vi "Initialise the Error log.vi"(8 "error in (no error)":errorcluster, 10 "Schema":string, 11 "Error Log in":refnum<class "Error Log.lvclass">) -> (0 "error out":errorcluster, 3 "Error Log out":refnum<class "Error Log.lvclass">)   [LabVIEW 2023, in "Data Analysis.lvlib" / "Error Log.lvlib" / "Error Log.lvclass"]
uses:
  Error Log.lvclass
  Error Log.lvclass/Error Log.ctl
  HardwareAbstractionLayer_LVOOP/Database/Database.lvclass
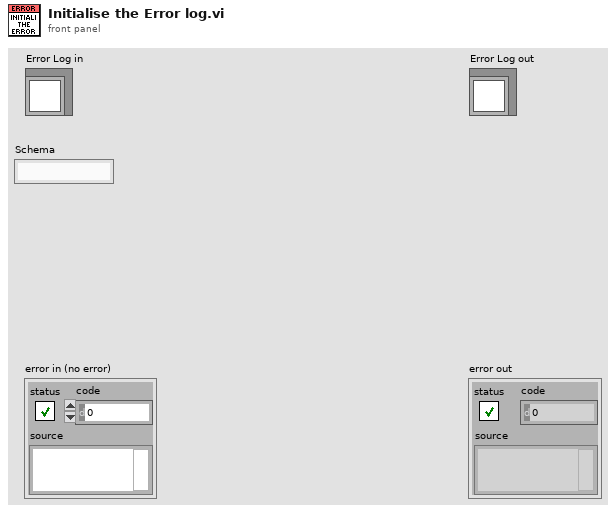
[diagram p1: front panel]
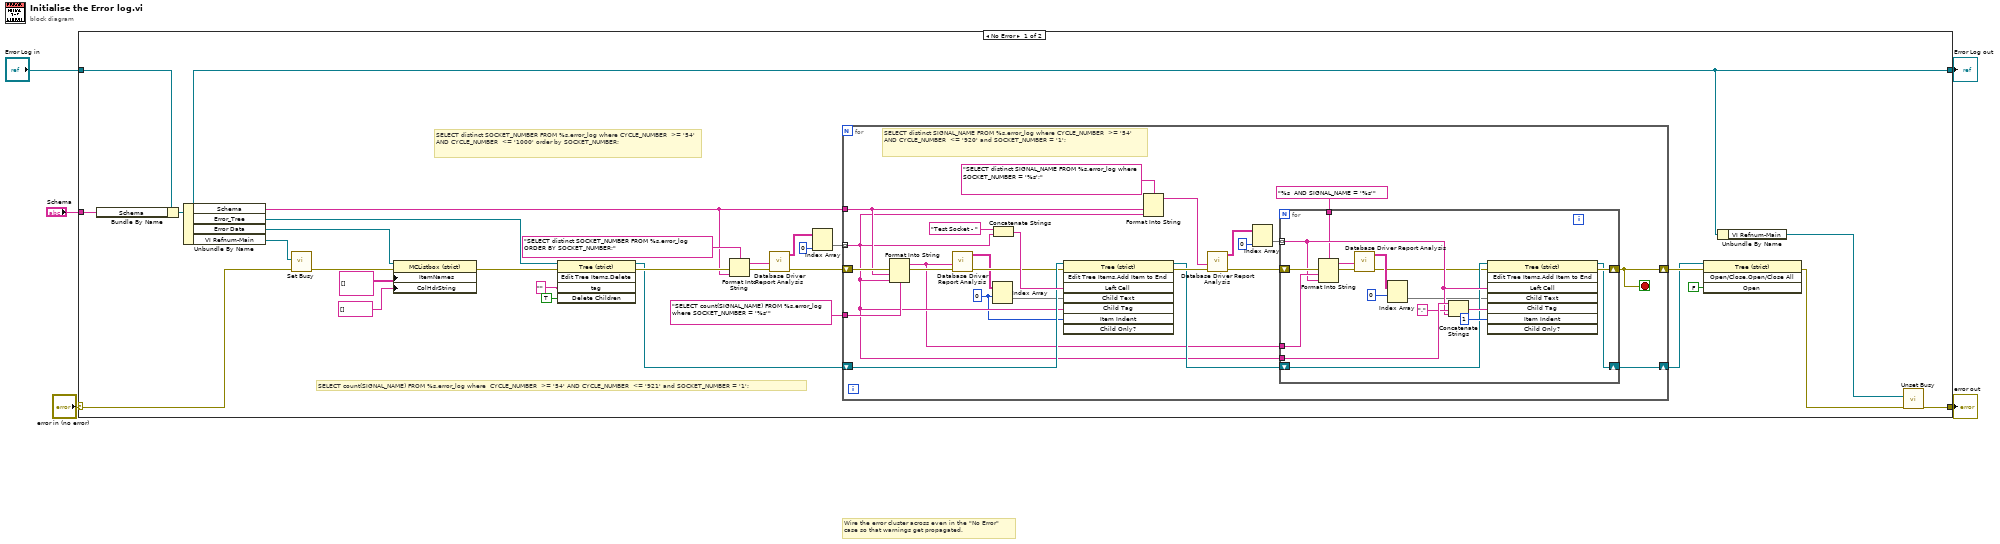
[diagram p0: block diagram]
diagram:
  # "Wire the error cluster across even in the \"No Error\"\ncase so that warnings get propagated."
  n1 = case shown="No Error" "error in (no error)" {
    selector: "error in (no error)" -> [w11 w78]
    tunnel: [w9 w77] -> w3
    tunnel: "Error Log in" -> [w19 w77]
    tunnel: "Schema" -> [w18 _]
    tunnel: [w6 w78] -> w1
    frame No Error {
      # "SELECT count(SIGNAL_NAME) FROM %s.error_log where  CYCLE_NUMBER  >= '54' AND CYCLE_NUMBER  <= '921' and SOCKET_NUMBER = '1';"
      # "SELECT distinct SOCKET_NUMBER FROM %s.error_log where CYCLE_NUMBER  >= '54' AND CYCLE_NUMBER  <= '1000' order by SOCKET_NUMBER;"
      n2 = Bundle By Name(cluster=w19, "Schema"=w18) -> (w9:refnum<class "Error Log.lvclass">)
      n3 = Unbundle By Name(w9) -> ("Schema"=w17:string, "Error_Tree"=w20:refnum<vi>, "Error Data"=w16:refnum<vi>, "VI Refnum-Main"=w12:refnum<vi>)
      n4 = call <vilib>:"Set Busy.vi"("error in (no error)"=w11, "VI reference (current VI)"=w12) -> ("error out"=w10:errorcluster)  [unwired: 8 in, 1 out]
      n5 = property class="MCListbox (strict)"(reference=w16, error in=w10, "ItemNames"=string[][] [] ("Item Names"), "ColHdrString"=string[] [] ("Column Header Strings[]")) -> (error out=w13:errorcluster)  [unwired: 1 out]
      n6 = invoke on="Invoke Node" class="Tree (strict)" method="Edit Tree Items.Delete"(reference=w20, error in=w13, "tag"="" ("Tag"), "Delete Children"=TRUE ("Delete Children?")) -> (reference out=w21:refnum<vi>, error out=w33:errorcluster)  [unwired: 1 in, 3 out]
      n7 = Format Into String(format string="SELECT distinct SOCKET_NUMBER FROM %s.error_log ORDER BY SOCKET_NUMBER;" ("SQL query"), error in=w33, w17) -> (resulting string=w30:string, error out=w34:errorcluster)  [unwired: 1 in]
      n8 = call "Database Driver Report Analysis.vi"("error in"=w34, "SQL query"=w30) -> ("error out"=w26:errorcluster, "data"=w27:string[][])  [unwired: 6 in, 2 out]
      n9 = Index Array(array=w27, index (col)=0 ("disabled index (col)")) -> (element=w28:string[])  [unwired: 1 in]
      n10 = for {
        tunnel: w28 -> [w41] mode=indexing
        shift-right: [w57] -> w35
        shift-left: w26 -> [w45]
        tunnel: w17 -> [w42]
        shift-right: [w47] -> w23
        shift-left: w21 -> [w49]
        tunnel: "SELECT count(SIGNAL_NAME) FROM %s.error_log where SOCKET_NUMBER = '%s'" ("SQL query") -> [w43]
        stop <- w57 stop-if-true
        w38 = 0 ("index (row)")
        # "SELECT distinct SIGNAL_NAME FROM %s.error_log where CYCLE_NUMBER  >= '54' AND CYCLE_NUMBER  <= '920' and SOCKET_NUMBER = '1';"
        n11 = Format Into String(format string=w43, error in=w45, w42, w41) -> (resulting string=w37:string, error out=w44:errorcluster)  [unwired: 1 in]
        n12 = call "Database Driver Report Analysis.vi"("error in"=w44, "SQL query"=w37) -> ("error out"=w46:errorcluster, "data"=w40:string[][])  [unwired: 6 in, 2 out]
        n13 = Index Array(array=w40, index (row)=w38) -> (element=w39:string[])  [unwired: 1 in]
        n14 = Concatenate Strings("Test Socket - " ("element"), w41) -> (w58:string)
        n15 = invoke on="Invoke Node" class="Tree (strict)" method="Edit Tree Items.Add Item to End"(reference=w49, error in=w46, "Left Cell"=w58, "Child Text"=w39, "Child Tag"=w41, "Item Indent"=w38) -> (reference out=w48:refnum<vi>, error out=w56:errorcluster)  [unwired: 2 in, 6 out]
        n16 = Format Into String(format string="SELECT distinct SIGNAL_NAME FROM %s.error_log where SOCKET_NUMBER = '%s';" ("SQL query"), w42, w41) -> (resulting string=w53:string)  [unwired: 2 in, 1 out]
        n17 = call "Database Driver Report Analysis.vi"("error in"=w56, "SQL query"=w53) -> ("error out"=w55:errorcluster, "data"=w51:string[][])  [unwired: 6 in, 2 out]
        n18 = Index Array(array=w51, index (col)=0 ("disabled index (col)")) -> (element=w50:string[])  [unwired: 1 in]
        n19 = for {
          shift-right: [w76] -> w57
          shift-left: w55 -> [w70]
          tunnel: w50 -> [w68] mode=indexing
          tunnel: w41 -> [w74]
          shift-right: [w71] -> w47
          shift-left: w48 -> [w66]
          tunnel: w37 -> [w69]
          tunnel: "%s  AND SIGNAL_NAME = '%s'" ("format string") -> [w67]
          n20 = Format Into String(format string=w67, error in=w70, w69, w68) -> (resulting string=w60:string, error out=w63:errorcluster)  [unwired: 1 in]
          n21 = call "Database Driver Report Analysis.vi"("error in"=w63, "SQL query"=w60) -> ("error out"=w62:errorcluster, "data"=w65:string[][])  [unwired: 6 in, 2 out]
          n22 = Index Array(array=w65, index (row)=0) -> (element=w61:string[])  [unwired: 1 in]
          n23 = Concatenate Strings(w74, "." ("string"), w68) -> (w72:string)
          n24 = invoke on="Invoke Node" class="Tree (strict)" method="Edit Tree Items.Add Item to End"(reference=w66, error in=w62, "Left Cell"=w68, "Child Text"=w61, "Child Tag"=w72, "Item Indent"=1 ("New Item Indentation")) -> (reference out=w71:refnum<vi>, error out=w76:errorcluster)  [unwired: 2 in, 6 out]
        }
      }
      n25 = invoke on="Invoke Node" class="Tree (strict)" method="Open/Close.Open/Close All"(reference=w23, error in=w35, "Open"=FALSE ("Open?")) -> (error out=w7:errorcluster)  [unwired: 1 in, 3 out]
      n26 = Unbundle By Name(w9) -> ("VI Refnum-Main"=w8:refnum<vi>)
      n27 = call <vilib>:"Unset Busy.vi"("error in (no error)"=w7, "VI reference (current VI)"=w8) -> ("error out"=w6:errorcluster)  [unwired: 9 in]
    }
    frame Error {
    }
  }
  "error out" <- w1
  "Error Log out" <- w3
